vi "Wench.vi"(11 "output cluster":T1) -> ()   [LabVIEW 2016]
uses:
  References/Refnums.vi
  Joystick/ControlsToCommands.ctl
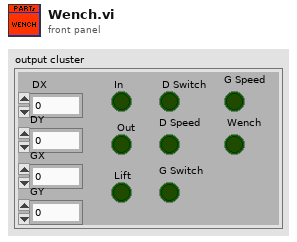
[diagram p1: front panel]
types:
  T1 = typedef "ControlsToCommands.ctl" = cluster{"DX":dbl, "DY":dbl, "GX":dbl, "GY":dbl, "In":bool, " Out":bool, "Lift":bool, "D Switch":bool, "D Speed":bool, "G Switch":bool, "G Speed":bool, " Wench":bool}
  T2 = typedef "WPI_MotorControlDeviceRef.ctl" = cluster{"DeviceStatus":errorcluster, "Type":T3, "PWM":cluster{"PWM Channel":T4, "DeadBand":T5}, "CAN":cluster{"Device Number":u8, "SetOutput VI Ref":variant, "GetOutput VI Ref":variant, "Enable VI Ref":variant, "Disable VI Ref":variant, "Data":variant}, "Invert":bool}
  T3 = typedef "WPI_MotorControlType.ctl" = enum16{"PWM", "CAN"}
  T4 = typedef "FPGA_DIOPWMChannel.ctl" = enum8{"PWM 0", "PWM 1", "PWM 2", "PWM 3", "PWM 4", "PWM 5", "PWM 6", "PWM 7", "PWM 8", "PWM 9", "PWM MXP 0", "PWM MXP 1", "PWM MXP 2", "PWM MXP 3", "PWM MXP 4", "PWM MXP 5", "PWM MXP 6", "PWM MXP 7", "PWM MXP 8", "PWM MXP 9", "Invalid"}
  T5 = typedef "WPI_PWMDeadband.ctl" = cluster{"Name":string, "maxPositivePwm":i32, "minPositivePwm":i32, "centerPwm":i32, "maxNegativePwm":i32, "minNegativePwm":i32, "angularRange":u16}
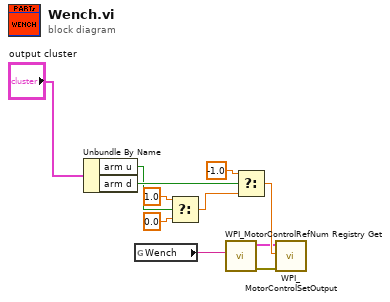
[diagram p0: block diagram]
diagram:
  n1 = Unbundle By Name("output cluster") -> ("arm u"=w5:bool, "arm d"=w6:bool)
  n2 = global read "Refnums.vi" "Wench"() -> (w4:string)
  n3 = Select(t=1.0, s=w5, f=0.0) -> (s? t:f=w9:dbl)
  n4 = call <vilib>:"WPI_MotorControlRefNum Registry Get.vi"("refnum name"=w4) -> ("error out"=w2:errorcluster, "MotorControlDevRef"=w3:T2)  [unwired: 9 in]
  n5 = Select(t=-1.0, s=w6, f=w9) -> (s? t:f=w10:dbl)
  n6 = call <vilib>:"WPI_MotorControlSetOutput.vi"("error in (no error)"=w2, "Output"=w10, "MotorControlDevRef"=w3) -> ()  [unwired: 6 in, 3 out]
